vi "Control Channels.vi"(8 "error in (no error)":errorcluster, 10 "Values":dbl[](array[numeric]), 11 "IVI Refnum in":refnum<k15>) -> (0 "error out":errorcluster, 3 "IVI Refnum out":refnum<k15>)   [LabVIEW 2020, in "PXI-2510 Engine.lvlib"]
uses:
  PXI-2510 Engine.lvlib
  <instrlib>/niSwitch/niSwitch.llb/niSwitch Relay Action.ctl
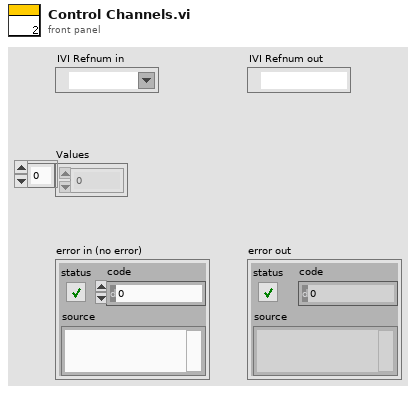
[diagram p1: front panel]
types:
  T1 = enum16{"Default", "DUT Pass Through", "DUT Open", "DUT Pass Through and FB A", "DUT Pass Through and FB B", "DUT FB A", "DUT FB B"}
  T2 = typedef "niSwitch Relay Action.ctl" = i32
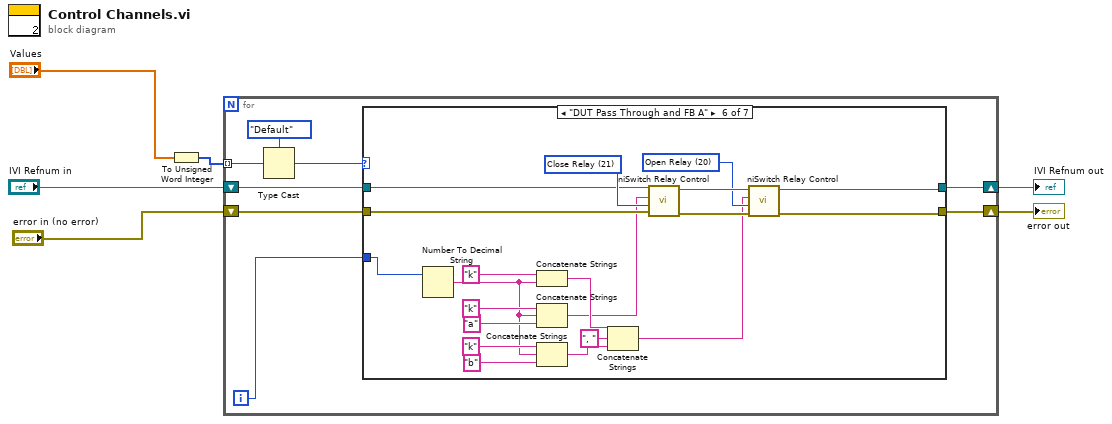
[diagram p0: block diagram]
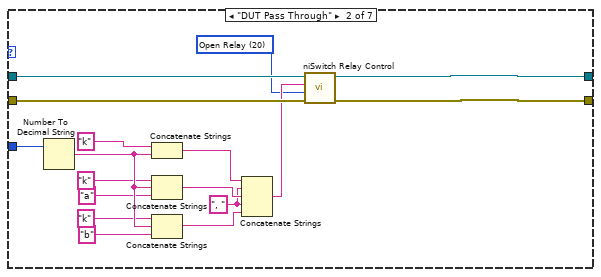
[diagram p3: hidden frame]
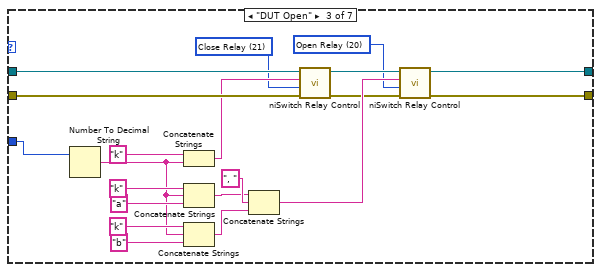
[diagram p4: hidden frame]
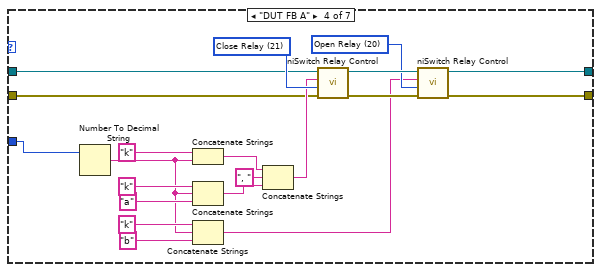
[diagram p5: hidden frame]
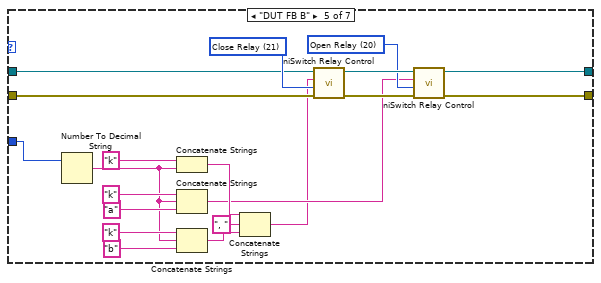
[diagram p6: hidden frame]
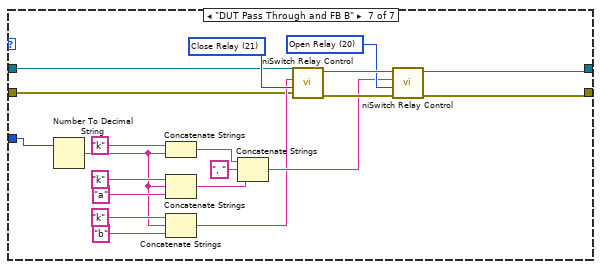
[diagram p7: hidden frame]
diagram:
  n1 = To Unsigned Word Integer(number="Values") -> (unsigned 16bit integer=w2:u16[])
  n2 = for {
    shift-right: [w12] -> w4
    shift-left: "IVI Refnum in" -> [w14]
    shift-right: [w11] -> w5
    shift-left: "error in (no error)" -> [w13]
    tunnel: w2 -> [w8] mode=indexing
    i -> [w7]
    n3 = Type Cast(type=T1."Default", x=w8) -> (*(type *) &x=w9:T1)
    n4 = case shown="\"DUT Pass Through and FB A\"" w9 {
      tunnel: w14 -> [w16 w33 w43 w59 w79 w100 w117]
      tunnel: w13 -> [w15 w32 w42 w55 w78 w98 w115]
      tunnel: [w16 w18 w34 w58 w76 w99 w116] -> w12
      tunnel: [w15 w17 w35 w54 w77 w97 w114] -> w11
      tunnel: w7 -> [_ w23 w44 w64 w84 w105 w124]
      frame "Default", Default {
      }
      frame "DUT Pass Through" {
        w19 = T2 20 items=["Open Relay"=20, "Close Relay"=21] ("relay action (Close Relay)")
        w21 = ", " ("string")
        n5 = Number To Decimal String(number=w23) -> (decimal integer string=w31:string)  [unwired: 1 in]
        n6 = Concatenate Strings("k", w31) -> (w22:string)
        n7 = Concatenate Strings("k", w31, "a") -> (w25:string)
        n8 = Concatenate Strings("k", w31, "b") -> (w24:string)
        n9 = Concatenate Strings(w22, w21, w25, w21, w24) -> (w20:string)
        n10 = call <instrlib>:"niSwitch Relay Control.vi"("error in (no error)"=w32, "relay action (Close Relay)"=w19, "relay names"=w20, "instrument handle"=w33) -> ("error out"=w17:errorcluster, "instrument handle out"=w18:refnum<k15>)  [unwired: 6 in]
      }
      frame "DUT Open" {
        w36 = T2 20 items=["Open Relay"=20, "Close Relay"=21] ("relay action (Close Relay)")
        w37 = T2 21 items=["Open Relay"=20, "Close Relay"=21] ("relay action (Close Relay)")
        n11 = Number To Decimal String(number=w44) -> (decimal integer string=w45:string)  [unwired: 1 in]
        n12 = Concatenate Strings("k", w45) -> (w38:string)
        n13 = Concatenate Strings("k", w45, "a") -> (w47:string)
        n14 = Concatenate Strings("k", w45, "b") -> (w46:string)
        n15 = Concatenate Strings(w47, ", " ("string"), w46) -> (w41:string)
        n16 = call <instrlib>:"niSwitch Relay Control.vi"("error in (no error)"=w42, "relay action (Close Relay)"=w37, "relay names"=w38, "instrument handle"=w43) -> ("error out"=w39:errorcluster, "instrument handle out"=w40:refnum<k15>)  [unwired: 6 in]
        n17 = call <instrlib>:"niSwitch Relay Control.vi"("error in (no error)"=w39, "relay action (Close Relay)"=w36, "relay names"=w41, "instrument handle"=w40) -> ("error out"=w35:errorcluster, "instrument handle out"=w34:refnum<k15>)  [unwired: 6 in]
      }
      frame "DUT FB A" {
        w60 = T2 20 items=["Open Relay"=20, "Close Relay"=21] ("relay action (Close Relay)")
        w61 = T2 21 items=["Open Relay"=20, "Close Relay"=21] ("relay action (Close Relay)")
        n18 = Number To Decimal String(number=w64) -> (decimal integer string=w67:string)  [unwired: 1 in]
        n19 = Concatenate Strings("k", w67) -> (w66:string)
        n20 = Concatenate Strings("k", w67, "a") -> (w65:string)
        n21 = Concatenate Strings("k", w67, "b") -> (w57:string)
        n22 = Concatenate Strings(w66, ", " ("string"), w65) -> (w56:string)
        n23 = call <instrlib>:"niSwitch Relay Control.vi"("error in (no error)"=w55, "relay action (Close Relay)"=w61, "relay names"=w56, "instrument handle"=w59) -> ("error out"=w62:errorcluster, "instrument handle out"=w63:refnum<k15>)  [unwired: 6 in]
        n24 = call <instrlib>:"niSwitch Relay Control.vi"("error in (no error)"=w62, "relay action (Close Relay)"=w60, "relay names"=w57, "instrument handle"=w63) -> ("error out"=w54:errorcluster, "instrument handle out"=w58:refnum<k15>)  [unwired: 6 in]
      }
      frame "DUT FB B" {
        w80 = T2 20 items=["Open Relay"=20, "Close Relay"=21] ("relay action (Close Relay)")
        w81 = T2 21 items=["Open Relay"=20, "Close Relay"=21] ("relay action (Close Relay)")
        n25 = Number To Decimal String(number=w84) -> (decimal integer string=w87:string)  [unwired: 1 in]
        n26 = Concatenate Strings("k", w87) -> (w86:string)
        n27 = Concatenate Strings("k", w87, "a") -> (w75:string)
        n28 = Concatenate Strings("k", w87, "b") -> (w85:string)
        n29 = Concatenate Strings(w86, ", " ("string"), w85) -> (w74:string)
        n30 = call <instrlib>:"niSwitch Relay Control.vi"("error in (no error)"=w78, "relay action (Close Relay)"=w81, "relay names"=w74, "instrument handle"=w79) -> ("error out"=w82:errorcluster, "instrument handle out"=w83:refnum<k15>)  [unwired: 6 in]
        n31 = call <instrlib>:"niSwitch Relay Control.vi"("error in (no error)"=w82, "relay action (Close Relay)"=w80, "relay names"=w75, "instrument handle"=w83) -> ("error out"=w77:errorcluster, "instrument handle out"=w76:refnum<k15>)  [unwired: 6 in]
      }
      frame "DUT Pass Through and FB A" {
        w101 = T2 20 items=["Open Relay"=20, "Close Relay"=21] ("relay action (Close Relay)")
        w102 = T2 21 items=["Open Relay"=20, "Close Relay"=21] ("relay action (Close Relay)")
        n32 = Number To Decimal String(number=w105) -> (decimal integer string=w108:string)  [unwired: 1 in]
        n33 = Concatenate Strings("k", w108) -> (w107:string)
        n34 = Concatenate Strings("k", w108, "a") -> (w95:string)
        n35 = Concatenate Strings("k", w108, "b") -> (w106:string)
        n36 = Concatenate Strings(w107, ", " ("string"), w106) -> (w96:string)
        n37 = call <instrlib>:"niSwitch Relay Control.vi"("error in (no error)"=w98, "relay action (Close Relay)"=w102, "relay names"=w95, "instrument handle"=w100) -> ("error out"=w103:errorcluster, "instrument handle out"=w104:refnum<k15>)  [unwired: 6 in]
        n38 = call <instrlib>:"niSwitch Relay Control.vi"("error in (no error)"=w103, "relay action (Close Relay)"=w101, "relay names"=w96, "instrument handle"=w104) -> ("error out"=w97:errorcluster, "instrument handle out"=w99:refnum<k15>)  [unwired: 6 in]
      }
      frame "DUT Pass Through and FB B" {
        w120 = T2 20 items=["Open Relay"=20, "Close Relay"=21] ("relay action (Close Relay)")
        w121 = T2 21 items=["Open Relay"=20, "Close Relay"=21] ("relay action (Close Relay)")
        n39 = Number To Decimal String(number=w124) -> (decimal integer string=w127:string)  [unwired: 1 in]
        n40 = Concatenate Strings("k", w127) -> (w126:string)
        n41 = Concatenate Strings("k", w127, "a") -> (w125:string)
        n42 = Concatenate Strings("k", w127, "b") -> (w118:string)
        n43 = Concatenate Strings(w126, ", " ("string"), w125) -> (w119:string)
        n44 = call <instrlib>:"niSwitch Relay Control.vi"("error in (no error)"=w115, "relay action (Close Relay)"=w121, "relay names"=w118, "instrument handle"=w117) -> ("error out"=w122:errorcluster, "instrument handle out"=w123:refnum<k15>)  [unwired: 6 in]
        n45 = call <instrlib>:"niSwitch Relay Control.vi"("error in (no error)"=w122, "relay action (Close Relay)"=w120, "relay names"=w119, "instrument handle"=w123) -> ("error out"=w114:errorcluster, "instrument handle out"=w116:refnum<k15>)  [unwired: 6 in]
      }
    }
  }
  "error out" <- w5
  "IVI Refnum out" <- w4
